vi "Test RFC3339.vi"(8 "error in":errorcluster) -> (0 "error out":errorcluster)   [LabVIEW 2013]
uses:
  <vilib>/Utility/file.llb/Read From Spreadsheet File (string).vi
  <vilib>/addons/_JKI Toolkits/Caraya/classes/Assert/Assert True.vi
  <vilib>/addons/_JKI Toolkits/Caraya/classes/Test/Test.lvclass
  <vilib>/addons/_JKI Toolkits/Caraya/classes/Assert/Assert.lvclass
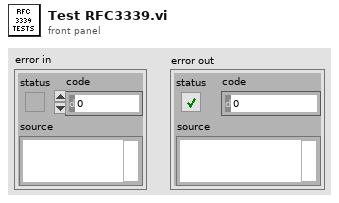
[diagram p1: front panel]
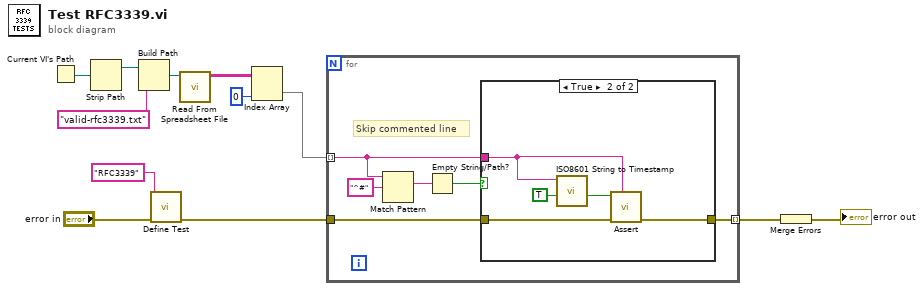
[diagram p0: block diagram]
diagram:
  n1 = Current VI's Path() -> (path=w6:path)
  n2 = Strip Path(path=w6) -> (stripped path=w7:path)  [unwired: 1 out]
  n3 = Build Path(base path=w7, name or relative path="valid-rfc3339.txt") -> (appended path=w8:path)
  n4 = call <vilib>:"Define Test.vi"("error in (no error)"="error in", "Label (VI Title)"="RFC3339") -> ("error out"=w12:errorcluster)  [unwired: 8 in, 1 out]
  n5 = call-poly <vilib>:"Read From Spreadsheet File.vi"("file path (dialog if empty)"=w8) -> ("all rows"=w3:string[][])  [unwired: 6 in, 4 out]
  n6 = Index Array(array=w3, index (col)=0 ("disabled index (col)")) -> (element=w5:string[])  [unwired: 1 in]
  n7 = for {
    tunnel: w5 -> [w16] mode=indexing
    tunnel: [w17] -> w9 mode=indexing
    tunnel: w12 -> [w18]
    # "Skip commented line"
    n8 = Match Pattern(string=w16, regular expression="^#") -> (match substring=w14:string)  [unwired: 1 in, 3 out]
    n9 = Empty String/Path?(string/path=w14) -> (empty?=w13:bool)
    n10 = case shown="True" w13 {
      tunnel: w18 -> [w19 w24]
      tunnel: [w19 w23] -> w17
      tunnel: w16 -> [_ w20]
      frame False {
        # "Skip"
      }
      frame True {
        n11 = call "ISO8601 String to Timestamp.vi"("Strict ISO? (T)"=TRUE, "ISO8601 String"=w20) -> ("valid?"=w21:bool)  [unwired: 7 in, 2 out]
        n12 = call-poly <vilib>:"Assert.vi"("Label"=w20, "error in (no error)"=w24, "True?"=w21) -> ("error out"=w23:errorcluster)  [unwired: 7 in, 1 out]
      }
    }
  }
  n13 = Merge Errors(w9) -> (→"error out":errorcluster)
